vi "Fetch Data Log.vi"(8 "error in (no error)":errorcluster {"code" format="%.0x"}, 9 "Data Log Type (1: Voltage)":i32(ring)=1 items=["Voltage"=1, "Current"=0], 10 "Channel Name (1)":string="1", 11 "VISA resource name":refnum<visa-resource-name>) -> (0 "error out":errorcluster {"code" format="%.0x"}, 1 "Peak to Peak":dbl format="%^.3e", 3 "VISA resource name out":refnum<visa-resource-name>)   [LabVIEW 2016, in "Agilent N6700 Series.lvlib"]
doc: "Returns the peak to peak value of the data logger between marker 1 and marker 2.\n\n<b>Note:</b>\nThis VI only applies to the N6705B and N6705C DC Power Analyzer."
uses:
  <instrlib>/Agilent N6700 Series/Agilent N6700 Series.lvlib
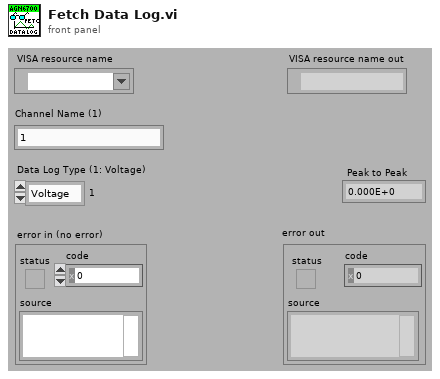
[diagram p1: front panel]
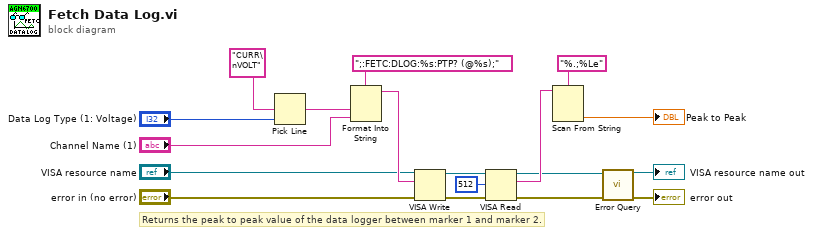
[diagram p0: block diagram]
diagram:
  # "Returns the peak to peak value of the data logger between marker 1 and marker 2."
  n1 = Pick Line(multi-line string="CURR\nVOLT", line index="Data Log Type (1: Voltage)") -> (output string=w10:string)  [unwired: 1 in]
  n2 = Format Into String(format string=";:FETC:DLOG:%s:PTP? (@%s);", w10, "Channel Name (1)") -> (resulting string=w16:string)  [unwired: 2 in, 1 out]
  n3 = VISA Write(VISA resource name="VISA resource name", write buffer=w16, error in (no error)="error in (no error)") -> (VISA resource name out=w8:refnum<visa-resource-name>, error out=w9:errorcluster)  [unwired: 1 out]
  n4 = VISA Read(VISA resource name=w8, byte count=u32 512, error in (no error)=w9) -> (VISA resource name out=w4:refnum<visa-resource-name>, read buffer=w13:string, error out=w5:errorcluster)  [unwired: 1 out]
  n5 = Scan From String(format string="%.;%Le", input string=w13) -> (output 1=→"Peak to Peak":dbl)  [unwired: 3 in, 3 out]
  n6 = call <instrlib>:"Error Query.vi"("VISA resource name"=w4, "error in (no error)"=w5) -> ("VISA resource name out"=→"VISA resource name out":refnum<visa-resource-name>, "error out"=→"error out":errorcluster)  [unwired: 10 in, 2 out]
